vi "RT Loop - UI Commands.vi"(11 "Message Queue":refnum<queue> caption="消息队列") -> ()   [LabVIEW 2013]
doc: "使用该模板构建简单状态机设计模式。各状态执行代码并决定转移状态。"
uses:
  support/Message Queue/Message Cluster.ctl
  controls/RT Loop - UI Communication State.ctl
  Globals/Global - Configuration Options.vi
  Globals/Global - RT Stream Connections.vi
  support/Message Queue/Message Queue.lvlib
  <resource>/objmgr/ni.dex.rc
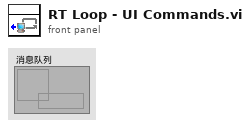
[diagram p1: front panel]
types:
  T1 = typedef "RT Loop - UI Communication State.ctl" = enum16{"Initialize", "Listen for UI Writer", "Receive UI Commands"}
  T2 = typedef "Message Queue.lvlib/Message Cluster.ctl" = cluster{"Message":string, "Message Data":variant}
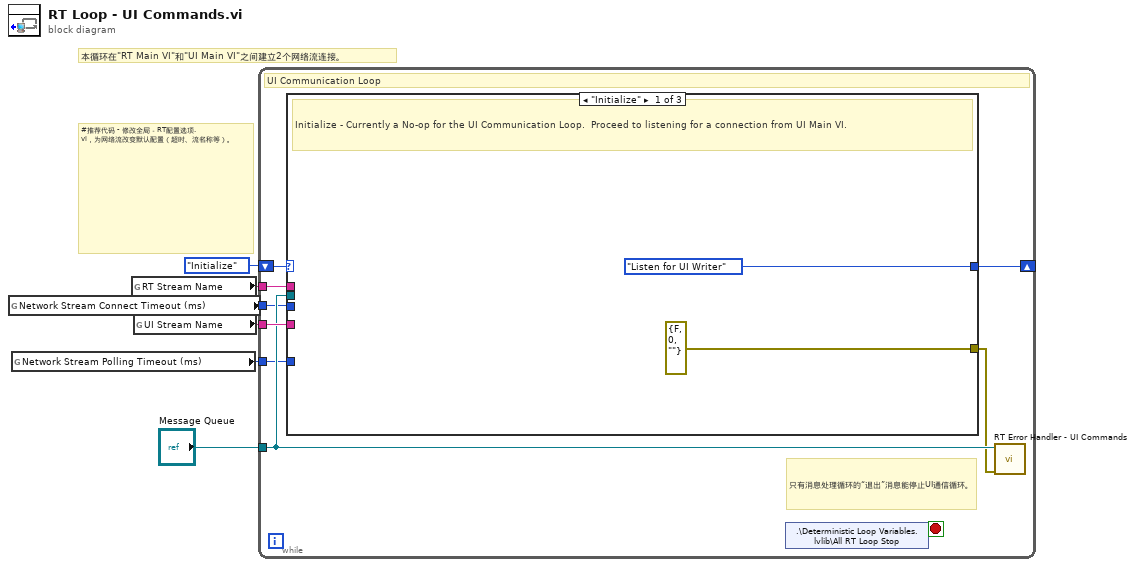
[diagram p0: block diagram]
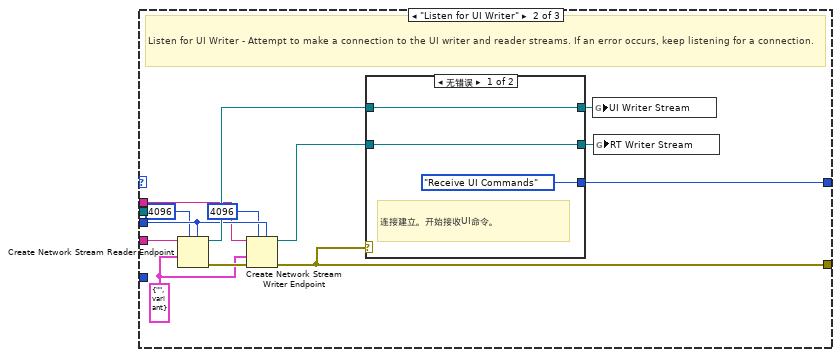
[diagram p2: hidden frame]
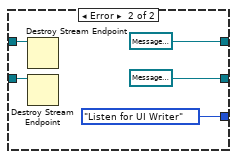
[diagram p3: hidden frame]
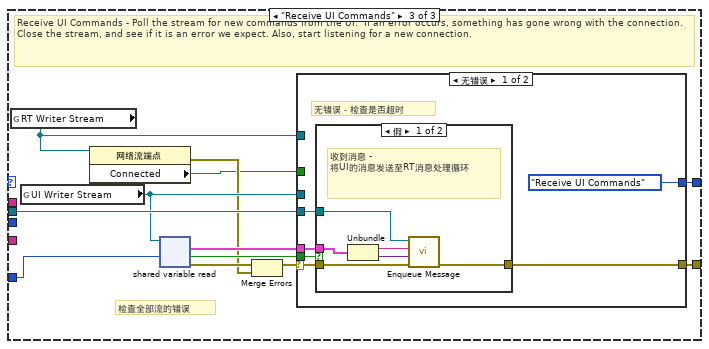
[diagram p4: hidden frame]
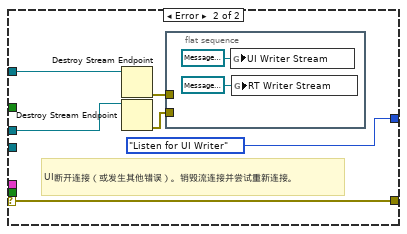
[diagram p6: hidden frame]
diagram:
  # "#推荐代码 - 修改全局－RT配置选项.vi，为网络流改变默认配置（超时、流名称等）。"
  # "本循环在\"RT Main VI\"和\"UI Main VI\"之间建立2个网络流连接。"
  n1 = global read "Global - Configuration Options.vi" "Network Stream Connect Timeout (ms)"() -> (w1:i32)
  n2 = global read "Global - Configuration Options.vi" "Network Stream Polling Timeout (ms)"() -> (w2:i32)
  n3 = global read "Global - Configuration Options.vi" "RT Stream Name"() -> (w3:string)
  n4 = global read "Global - Configuration Options.vi" "UI Stream Name"() -> (w4:string)
  n5 = while {
    shift-right: [w14] -> _
    shift-left: RT_Loop_-_UI_Communication_State."Initialize" ("RT Loop - Host Communication State") -> [w15]
    tunnel: "Message Queue" -> [w12]
    tunnel: w4 -> [w13]
    tunnel: w3 -> [w10]
    tunnel: w2 -> [w9]
    tunnel: w1 -> [w8]
    stop <- w7 stop-if-true
    # "只有消息处理循环的“退出”消息能停止UI通信循环。"
    # "UI Communication Loop"
    n6 = case shown="\"Initialize\"" w15 {
      tunnel: [RT_Loop_-_UI_Communication_State."Listen for UI Writer" ("RT Loop - Host Communication State") w29 w49] -> w14
      tunnel: [errorcluster {"status"=FALSE, "code"=0, "source"=""} ("error IO") w24 w50] -> w11
      tunnel: w8 -> [_ w23 _]
      tunnel: w13 -> [_ w28 _]
      tunnel: w12 -> [_ _ w48]
      tunnel: w10 -> [_ w22 _]
      tunnel: w9 -> [_ _ w39]
      frame "Initialize" {
        # "Initialize - Currently a No-op for the UI Communication Loop.  Proceed to listening for a connection from UI Main VI."
      }
      frame "Listen for UI Writer" {
        w26 = T2 {"Message"="", "Message Data"=variant} ("Message Cluster")
        # "Listen for UI Writer - Attempt to make a connection to the UI writer and reader streams. If an error occurs, keep listening for a connection."
        n7 = Create Network Stream Reader Endpoint(5:w23, 7:4096 ("reader buffer size"), 9:w26, 11:w28) -> (0:w27:errorcluster, 3:w30:refnum<k21>)  [unwired: 3 in]
        n8 = Create Network Stream Writer Endpoint(5:w23, 7:4096 ("writer buffer size"), 8:w27, 9:w26, 11:w22) -> (0:w24:errorcluster, 3:w25:refnum<k21>)  [unwired: 2 in]
        n9 = case shown="无错误" w24 {
          tunnel: w30 -> [w32 w35]
          tunnel: [RT_Loop_-_UI_Communication_State."Receive UI Commands" ("RT Loop - Host Communication State") RT_Loop_-_UI_Communication_State."Listen for UI Writer" ("RT Loop - Host Communication State")] -> w29
          tunnel: w25 -> [w31 w34]
          tunnel: [w32 refnum<k21> refnum] -> w21
          tunnel: [w31 refnum<k21> refnum] -> w20
          frame No Error {
            # "连接建立。开始接收UI命令。"
          }
          frame Error {
            n10 = Destroy Stream Endpoint(11:w35) -> ()  [unwired: 1 in, 1 out]
            n11 = Destroy Stream Endpoint(11:w34) -> ()  [unwired: 1 in, 1 out]
          }
        }
        n12 = global write "Global - RT Stream Connections.vi" "UI Writer Stream"(w21) -> ()
        n13 = global write "Global - RT Stream Connections.vi" "RT Writer Stream"(w20) -> ()
      }
      frame "Receive UI Commands" {
        # "检查全部流的错误"
        # "Receive UI Commands - Poll the stream for new commands from the UI.  If an error occurs, something has gone wrong with the connection. Close the stream, and see if it is an error we expect. Also, start listening for a new connection."
        n14 = global read "Global - RT Stream Connections.vi" "RT Writer Stream"() -> (w40:refnum<k21>)
        n15 = global read "Global - RT Stream Connections.vi" "UI Writer Stream"() -> (w44:refnum<k21>)
        n16 = property class="网络流端点"(reference=w40) -> (error out=w42:errorcluster, "Connected"=w41:bool)  [unwired: 1 in, 1 out]
        n17 = shared-variable-read(w44, w39) -> (w45:errorcluster, w46:bool, w47:T2)  [unwired: 1 in, 1 out]
        n18 = Merge Errors(w45, w42) -> (w43:errorcluster)
        n19 = case shown="无错误" w43 {
          selector: w43 -> [w54 w68]
          tunnel: [w53 w68] -> w50
          tunnel: w46 -> [w56 _]
          tunnel: w47 -> [w55 _]
          tunnel: [RT_Loop_-_UI_Communication_State."Receive UI Commands" ("RT Loop - Host Communication State") RT_Loop_-_UI_Communication_State."Listen for UI Writer" ("RT Loop - Host Communication State")] -> w49
          tunnel: w48 -> [w52 _]
          tunnel: w44 -> [_ w65]
          tunnel: w41 -> [_ _]
          tunnel: w40 -> [_ w64]
          frame No Error {
            # "无错误－检查是否超时"
            n20 = case shown="假" w56 {
              tunnel: w55 -> [w61 _]
              tunnel: w54 -> [w62 w63]
              tunnel: [w57 w63] -> w53
              tunnel: w52 -> [w58 _]
              frame False {
                # "收到消息 - 将UI的消息发送至RT消息处理循环"
                n21 = Unbundle(w61) -> ("Message"=w60:string, "Message Data"=w59:variant)
                n22 = call "Enqueue Message.vi"("error in (no error)"=w62, "Message Data"=w59, "Message"=w60, "Message Queue"=w58) -> ("error out"=w57:errorcluster)  [unwired: 6 in, 1 out]
              }
              frame True {
                # "超时－无新命令"
              }
            }
          }
          frame Error {
            # "UI断开连接（或发生其他错误）。销毁流连接并尝试重新连接。"
            n23 = Destroy Stream Endpoint(11:w64) -> (0:w67:errorcluster)  [unwired: 1 in]
            n24 = Destroy Stream Endpoint(11:w65) -> (0:w66:errorcluster)  [unwired: 1 in]
            n25 = flat-sequence {
              tunnel: w67 -> [_]
              tunnel: w66 -> [_]
              frame #0 {
                n26 = global write "Global - RT Stream Connections.vi" "UI Writer Stream"(refnum<k21> refnum ("Host Writer Stream")) -> ()
                n27 = global write "Global - RT Stream Connections.vi" "RT Writer Stream"(refnum<k21> refnum ("RT Writer Stream")) -> ()
              }
            }
          }
        }
      }
    }
    n28 = shared-variable ".\\Deterministic Loop Variables.lvlib\\All RT Loop Stop"() -> (w7:bool)  [unwired: 1 in, 1 out]
    n29 = call "RT Error Handler - UI Commands.vi"("error in (no error)"=w11, "Message Queue"=w12) -> ()  [unwired: 9 in, 1 out]
  }
